vi "example 12 - enums.vi"() -> ()   [LabVIEW 2020]
uses:
  ui-testing.lvlib
panel:
  out "Selected enum item":string
  in  "Enum":enum16{"a", "b", "c", "d", "e"}(ring)
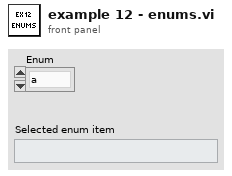
[diagram p1: front panel]
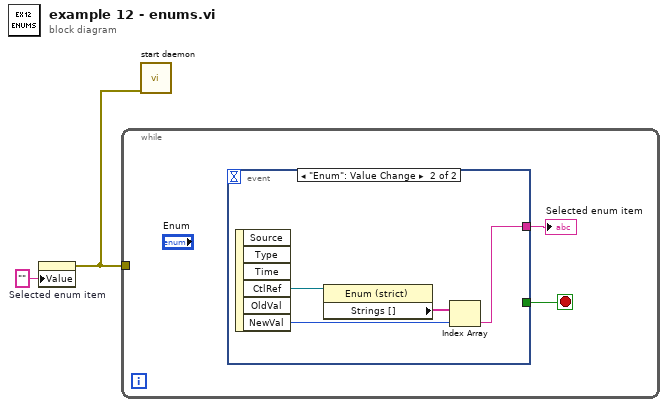
[diagram p0: block diagram]
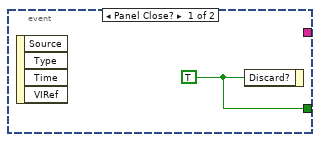
[diagram p2: hidden frame]
diagram:
  n1 = property on="Selected enum item" class="Str"("Value"="" ("Selected tab")) -> (error out=w1:errorcluster)  [unwired: 2 in, 1 out]
  n2 = while {
    tunnel: w1 -> [_]
    stop <- w4 stop-if-true
    n3 = event shown="[1] \"Enum\": Value Change" {
      selector: _ -> [_ _]
      dyn-events: _ -> [_ _]
      timeout: _ -> [_ _]
      tunnel: [w5 _] -> w4
      tunnel: [_ w6] -> w3
      event Panel Close? {
        w5 = TRUE
        n4 = event-data() -> ()  [unwired: 1 in, 4 out]
        n5 = event-data("Discard?"=w5) -> ()  [unwired: 1 in, 1 out]
      }
      event "Enum": Value Change {
        n6 = event-data() -> ("CtlRef"=w9:refnum<vi>, "NewVal"=w7:enum16{"a", "b", "c", "d", "e"})  [unwired: 1 in, 4 out]
        n7 = property class="Enum (strict)"(reference=w9) -> ("Strings []"=w8:string[])  [unwired: 1 in, 2 out]
        n8 = Index Array(array=w8, index=w7) -> (element=w6:string)
      }
    }
    "Selected enum item" <- w3
  }
  n9 = call "start daemon.vi"("error in (no error)"=w1) -> ()  [unwired: 10 in, 1 out]
